vi "SDKSID4_Close SID4.vi"(4 "error in (no error)":errorcluster, 7 "SDKSID4 session In":T1) -> (0 "error out":errorcluster, 3 "SDKSID4 session Out":T1)   [LabVIEW 2013]
doc: "This VI closes a OASys session. It aborts all pending measurements and releases memory devoted to the session."
uses:
  Refnum SDKSID4 session.ctl
  SID4_SDK.dll
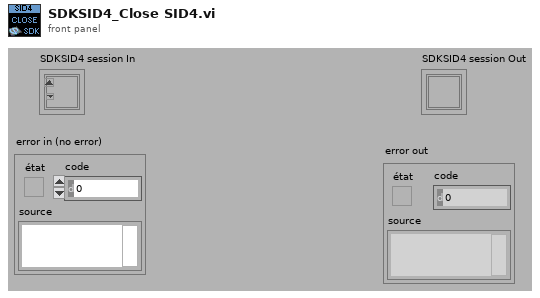
[diagram p1: front panel]
types:
  T1 = typedef "Refnum SDKSID4 session.ctl" = refnum<k1>
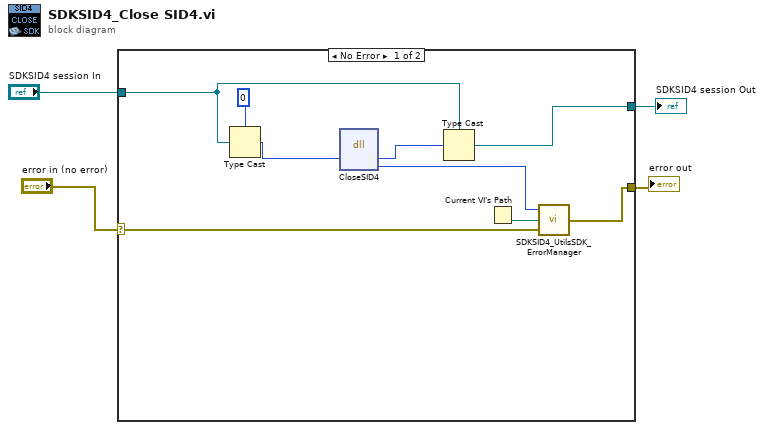
[diagram p0: block diagram]
diagram:
  n1 = case shown="No Error" "error in (no error)" {
    selector: "error in (no error)" -> [w5 w15]
    tunnel: [w6 w15] -> w4
    tunnel: "SDKSID4 session In" -> [w10 w14]
    tunnel: [w9 w14] -> w1
    frame No Error {
      n2 = Type Cast(type=u32 0, x=w10) -> (*(type *) &x=w12:u32)
      n3 = dll-call lib="C:/Program Files/SID4_SDK/DLL SDK/BIN/SID4_SDK.dll" fn="CloseSID4"("SID4SessionID"=w12) -> ("SID4SessionID"=w11:u32, "Error"=w7:i32)  [unwired: 5 in, 2 out]
      n4 = Type Cast(type=w10, x=w11) -> (*(type *) &x=w9:T1)
      n5 = Current VI's Path() -> (path=w8:path)
      n6 = call "SDKSID4_UtilsSDK_ErrorManager.vi"("error IN"=w5, "VI PathFile"=w8, "ErrorCode"=w7) -> ("error OUT"=w6:errorcluster)
    }
    frame Error {
    }
  }
  "error out" <- w4
  "SDKSID4 session Out" <- w1
